vi "ArtificialHorizon.vi"(8 "error in (no error)":errorcluster caption="Fehler (Eingang, kein Fehler)", 10 "SBG Data Cluster":T1) -> (0 "error out":errorcluster caption="Fehler (Ausgang)", 2 "ArtificialHorizon":picture)   [LabVIEW 2023]
uses:
  SBG Data Cluster.ctl
  <vilib>/Utility/miscctls.llb/LVBoundsTypeDef.ctl
  <vilib>/picture/picture.llb/imagedata.ctl
panel:
  out "GaugePicture":picture
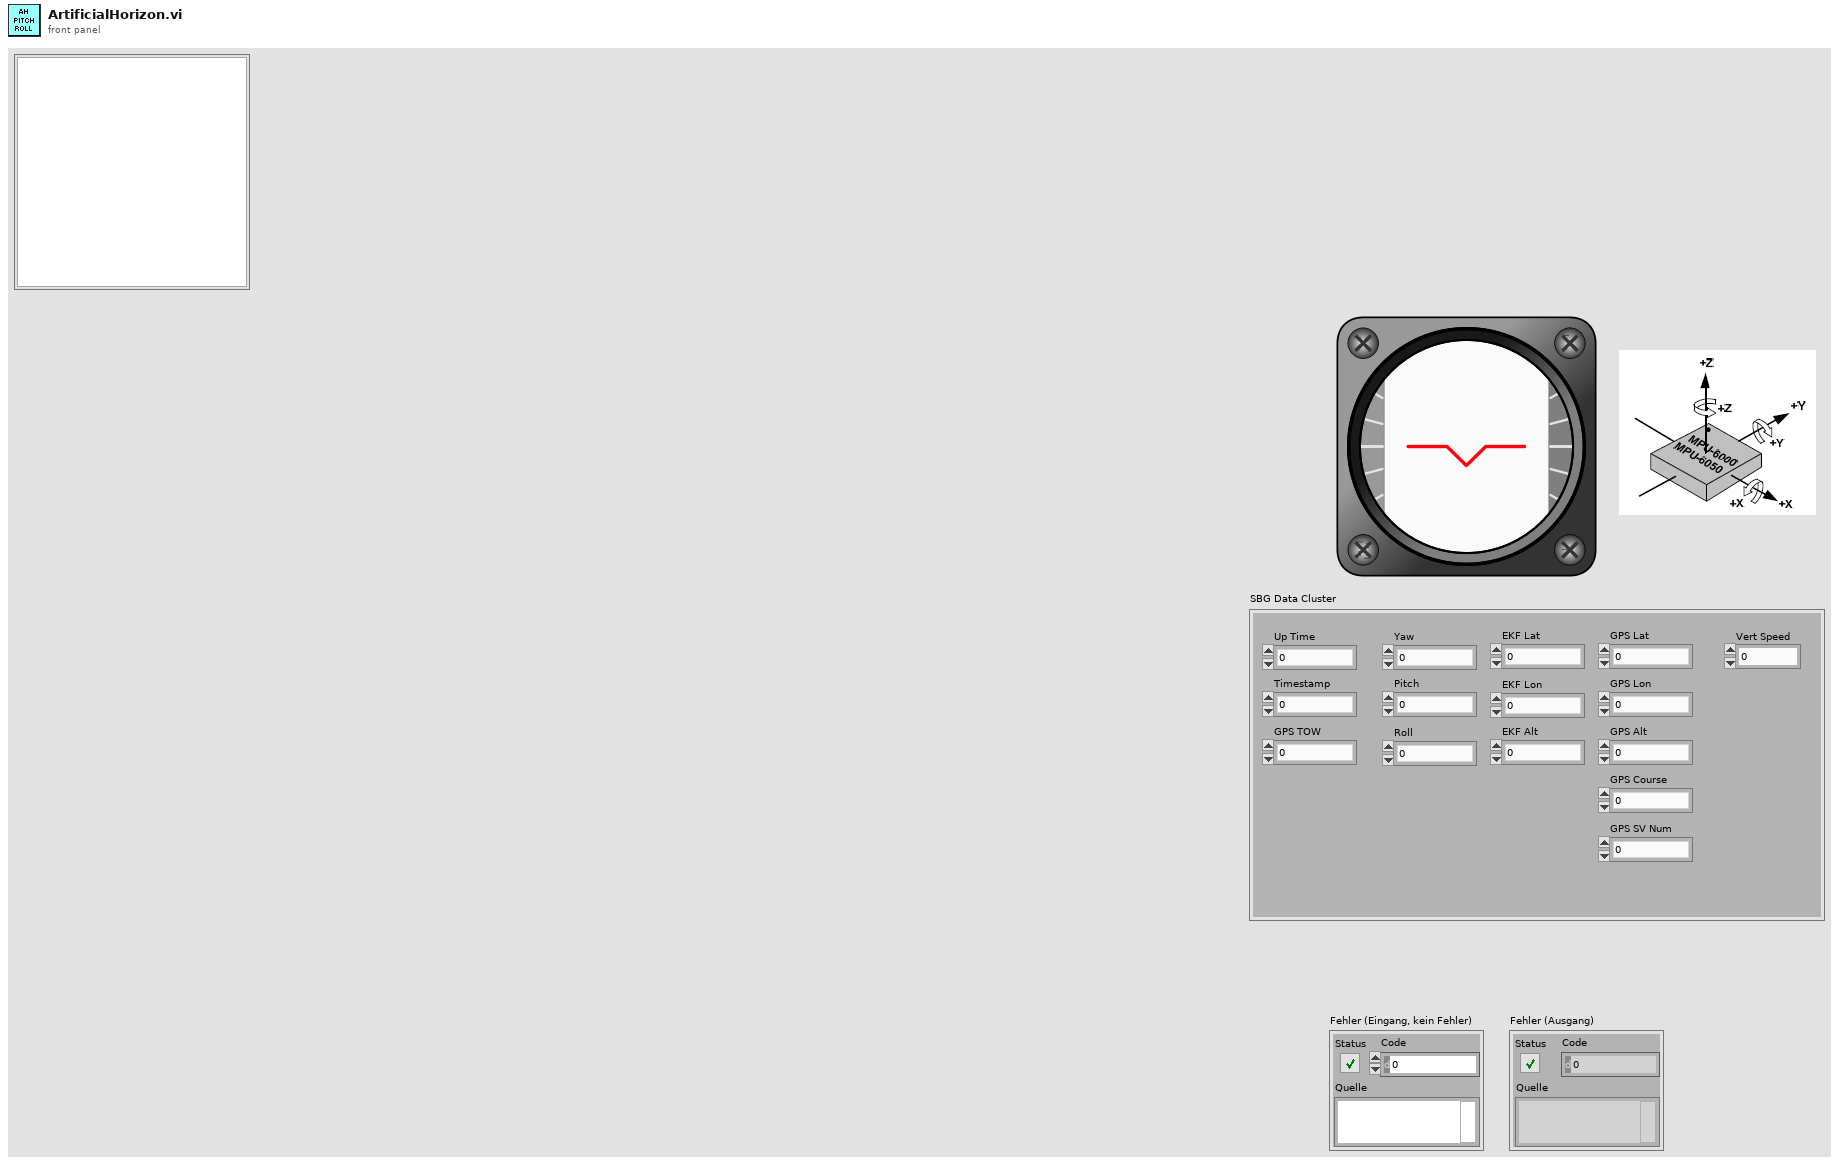
[diagram p1: front panel]
types:
  T1 = typedef "SBG Data Cluster.ctl" = cluster{"Up Time":u32, "Timestamp":u32, "Yaw":sgl, "Pitch":sgl, "Roll":sgl, "EKF Lat":dbl, "EKF Lon":dbl, "EKF Alt":dbl, "GPS Lat":dbl, "GPS Lon":dbl, "GPS Alt":dbl, "GPS Course":sgl, "GPS SV Num":u8, "GPS TOW":u32, "Vert Speed":dbl}
  T2 = typedef "LVBoundsTypeDef.ctl" = cluster{"Width":u32, "Height":u32}
  T3 = typedef "imagedata.ctl" = cluster{"image type":i32, "image depth":i32, "image":u8[], "mask":u8[], "colors":u32[], "Rectangle":cluster{"left":i16, "top":i16, "right":i16, "bottom":i16}}
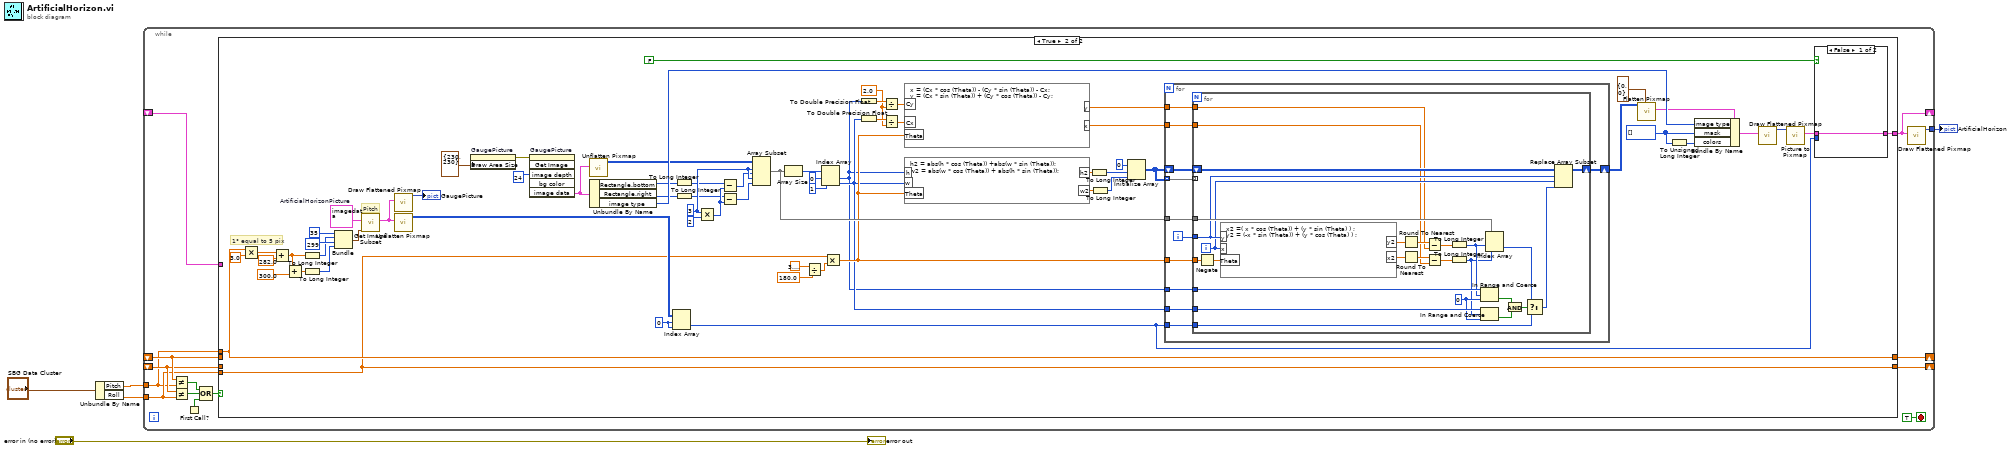
[diagram p0: block diagram]
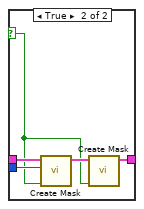
[diagram p3: hidden frame]
diagram:
  n1 = Unbundle By Name("SBG Data Cluster") -> ("Pitch"=w3:sgl, "Roll"=w2:sgl)
  n2 = while {
    shift-right: [w17] -> _
    shift-left: _ -> [w16]
    shift-right: [w13] -> _
    shift-left: _ -> [w12]
    tunnel: w2 -> [w8]
    shift-right: [w11] -> _
    shift-left: _ -> [w10]
    tunnel: w3 -> [w7]
    tunnel: [w6] -> w4
    stop <- TRUE stop-if-true
    n3 = Not Equal?(x=w16, y=w7) -> (x != y?=w19:bool)
    n4 = Not Equal?(x=w12, y=w8) -> (x != y?=w14:bool)
    n5 = First Call?() -> (First Call?: T/F=w15:bool)
    n6 = Compound Arithmetic op=OR(w19, w14, w15) -> (w18:bool)
    n7 = case shown="True" w18 {
      tunnel: w16 -> [w20 _]
      tunnel: [w22 w23] -> w11
      tunnel: [w20 w82] -> w17
      tunnel: w10 -> [w22 _]
      tunnel: w12 -> [w21 _]
      tunnel: [w21 w24] -> w13
      tunnel: w8 -> [_ w24]
      tunnel: w7 -> [_ w82]
      frame False {
      }
      frame True {
        w71 = 0 ("index (row)")
        w66 = u8[] [] ("mask")
        w61 = 3 ("Array Index")
        w42 = 2.0 ("y")
        w77 = T3 {"image type"=0, "image depth"=24, "image"=array[711900 elements], "mask"=[], "colors"=[], "Rectangle"={"left"=0, "top"=0, "right"=300, "bottom"=791}}  # ArtificialHorizonPicture
        # "Pitch"
        # "1° equal to 5 pix"
        n8 = Multiply(x=w82, y=3.0) -> (x*y=w88:dbl)
        n9 = Add(x=w88, y=282.0) -> (x+y=w79:dbl)
        n10 = Add(x=w79, y=300.0) -> (x+y=w85:dbl)
        n11 = To Long Integer(number=w79) -> (32bit integer=w81:i32)
        n12 = To Long Integer(number=w85) -> (32bit integer=w78:i32)
        n13 = Bundle(35, w81, 299, w78) -> (w83:cluster{i32, i32, i32, i32})  [unwired: 1 out]
        n14 = call <vilib>:"Get Image Subset.vi"("subset rect"=w83, "image data"=w77) -> ("image subset"=w25:T3)  [unwired: 5 out]
        n15 = call <vilib>:"Draw Flattened Pixmap.vi"("image data"=w25) -> ("new picture"=→"GaugePicture":picture)  [unwired: 1 in, 7 out]
        n16 = call <vilib>:"Unflatten Pixmap.vi"("image data"=w25) -> ("24-bit pixmap"=w75:u32[][])  [unwired: 4 in, 6 out]
        n17 = property on="GaugePicture" class="Pict"("Draw Area Size"=T2 {"Width"=230, "Height"=230} ("Größe des Darstellungsbereichs")) -> (error out=w50:errorcluster)  [unwired: 2 in, 1 out]
        n18 = invoke on="GaugePicture" class="Bild" method="Get Image"(error in=w50, "image depth"=24 ("Bildtiefe")) -> ("image data"=w52:T3)  [unwired: 4 in, 5 out]
        n19 = call <vilib>:"Unflatten Pixmap.vi"("image data"=w52) -> ("24-bit pixmap"=w72:u32[][])  [unwired: 4 in, 6 out]
        n20 = Unbundle By Name(w52) -> ("Rectangle.bottom"=w53:i16, "Rectangle.right"=w55:i16, "image type"=w74:i32)
        n21 = Index Array(array=w75, index (row)=w71, index (col)=w71) -> (element=w76:u32)
        n22 = To Long Integer(number=w53) -> (32bit integer=w54:i32)
        n23 = To Long Integer(number=w55) -> (32bit integer=w56:i32)
        n24 = Multiply(x=w61, y=2) -> (x*y=w60:i32)
        n25 = Subtract(x=w54, y=w60) -> (x-y=w57:i32)
        n26 = Subtract(x=w56, y=w60) -> (x-y=w58:i32)
        n27 = Array Subset(array=w72, index (row)=w61, length (row)=w57, index (col)=w61, length (col)=w58) -> (w62:u32[][])
        n28 = Array Size(array=w62) -> (size(s)=w33:i32[])
        n29 = Divide(x=3.141592653589793, y=180.0) -> (x/y=w28:dbl)
        n30 = Index Array(array=w33, index #1=0 ("Index"), index #2=1 ("Index")) -> (element #1=w45:i32, element #2=w46:i32)
        n31 = Multiply(x=w24, y=w28) -> (x*y=w47:dbl)
        n32 = To Double Precision Float(number=w45) -> (double precision float=w43:dbl)
        n33 = To Double Precision Float(number=w46) -> (double precision float=w44:dbl)
        n34 = Divide(x=w43, y=w42) -> (x/y=w41:dbl)
        n35 = Divide(x=w44, y=w42) -> (x/y=w40:dbl)
        n36 = formula code="x = (Cx * cos (Theta)) - (Cy * sin (Theta)) - Cx;\ny = (Cx * sin (Theta)) + (Cy * cos (Theta)) - Cy;"("Cx"=w40, "Cy"=w41, "Theta"=w47) -> ("x"=w48:dbl, "y"=w49:dbl)
        n37 = formula code="h2 = abs(h * cos (Theta)) +abs(w * sin (Theta)); \nw2 = abs(w * cos (Theta)) + abs(h * sin (Theta));"("h"=w45, "w"=w46, "Theta"=w47) -> ("h2"=w37:dbl, "w2"=w36:dbl)
        n38 = To Long Integer(number=w37) -> (32bit integer=w38:i32)
        n39 = To Long Integer(number=w36) -> (32bit integer=w39:i32)
        n40 = Initialize Array(u32 0, w38, w39) -> (w35:u32[][])
        n41 = for {
          tunnel: w62 -> [w106]
          tunnel: w47 -> [w101]
          shift-right: [w104] -> w64
          shift-left: w35 -> [w103]
          tunnel: w35 -> [w102] mode=indexing
          tunnel: w46 -> [w100]
          tunnel: w45 -> [w99]
          tunnel: w48 -> [w98]
          tunnel: w49 -> [w97]
          tunnel: w76 -> [w96]
          i -> [w105]
          n42 = for {
            tunnel: w106 -> [w127]
            tunnel: w105 -> [w125]
            tunnel: w101 -> [w128]
            shift-right: [w130] -> w104
            shift-left: w103 -> [w129]
            tunnel: w102 -> [_] mode=indexing
            tunnel: w100 -> [w120]
            tunnel: w99 -> [w121]
            tunnel: w98 -> [w112]
            tunnel: w97 -> [w111]
            tunnel: w96 -> [w109]
            i -> [w124]
            w110 = 0 ("lower limit")
            n43 = Negate(x=w128) -> (-x=w126:dbl)
            n44 = formula code="x2 =( x * cos (Theta)) + (y * sin (Theta) ) ;\ny2 = (-x * sin (Theta)) + (y * cos (Theta) ) ;"("y"=w125, "x"=w124, "Theta"=w126) -> ("y2"=w132:dbl, "x2"=w131:dbl)
            n45 = Round To Nearest(number=w132) -> (nearest integer value=w123:dbl)
            n46 = Round To Nearest(number=w131) -> (nearest integer value=w122:dbl)
            n47 = Subtract(x=w123, y=w111) -> (x-y=w118:dbl)
            n48 = Subtract(x=w122, y=w112) -> (x-y=w119:dbl)
            n49 = To Long Integer(number=w118) -> (32bit integer=w108:i32)
            n50 = To Long Integer(number=w119) -> (32bit integer=w107:i32)
            n51 = In Range and Coerce(upper limit=w121, x=w108, lower limit=w110) -> (In Range?=w116:bool)  [unwired: 1 out]
            n52 = In Range and Coerce(upper limit=w120, x=w107, lower limit=w110) -> (In Range?=w115:bool)  [unwired: 1 out]
            n53 = Index Array(array=w127, index (row)=w108, index (col)=w107) -> (element=w117:u32)
            n54 = And(x=w116, y=w115) -> (x .and. y?=w114:bool)
            n55 = Select(t=w117, s=w114, f=w109) -> (s? t:f=w113:u32)
            n56 = Replace Array Subset(array=w129, new element=w113, index (row)=w125, index (col)=w124) -> (w130:u32[][])
          }
        }
        n57 = call <vilib>:"Flatten Pixmap.vi"("top left"=cluster{"x":i16, "y":i16} {"x"=0, "y"=0}, "24-bit pixmap"=w64) -> ("image data"=w65:T3)  [unwired: 9 in]
        n58 = To Unsigned Long Integer(number=w66) -> (unsigned 32bit integer=w67:u32[])
        n59 = Bundle By Name(cluster=w65, "image type"=w74, "mask"=w66, "colors"=w67) -> (w68:T3)
        n60 = call <vilib>:"Draw Flattened Pixmap.vi"("image data"=w68) -> ("new picture"=w69:picture)  [unwired: 8 in]
        n61 = call <vilib>:"Picture to Pixmap.vi"("picture"=w69) -> ("image data"=w73:T3)  [unwired: 3 in, 7 out]
        n62 = case shown="False" FALSE ("Maske kombinieren? (F)") {
          selector: FALSE ("Maske kombinieren? (F)") -> [_ w91]
          tunnel: w73 -> [w90 w95]
          tunnel: [w90 w93] -> w23
          tunnel: w76 -> [_ w92]
          frame False {
          }
          frame True {
            n63 = call <vilib>:"Create Mask.vi"("Combine Masks? (F)"=w91, "Mask Color (Black)"=w92, "image data"=w95) -> ("image data"=w94:T3)  [unwired: 1 in, 7 out]
            n64 = call <vilib>:"Create Mask.vi"("Combine Masks? (F)"=w91, "image data"=w94) -> ("image data"=w93:T3)  [unwired: 2 in, 7 out]
          }
        }
      }
    }
    n65 = call <vilib>:"Draw Flattened Pixmap.vi"("image data"=w11) -> ("new picture"=w6:picture)  [unwired: 1 in, 7 out]
  }
  "ArtificialHorizon" <- w4
  "error out" <- "error in (no error)"
